vi "ReadCA.vi"(0 "CA":T2(array[cluster]), 1 "Index":u32) -> (7 "square":T1)   [LabVIEW 2020]
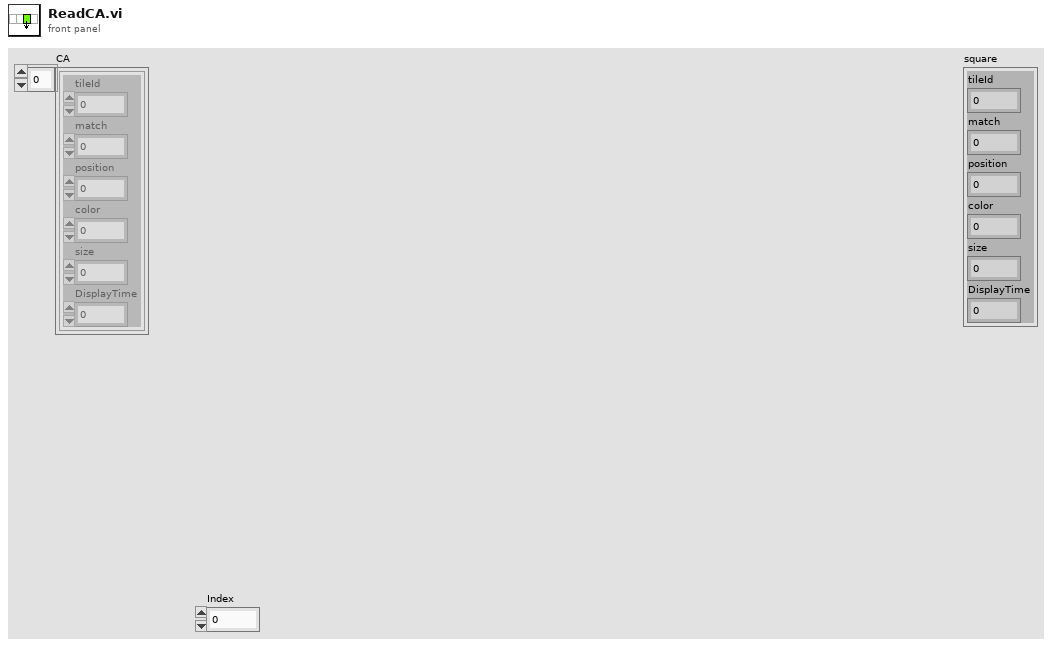
[diagram p1: front panel]
types:
  T1 = cluster{"tileId":i32, "match":i32, "position":i32, "color":u32, "size":i32, "DisplayTime":i32}
  T2 = cluster{"tileId":i32, "match":i32, "position":i32, "color":u32, "size":i32, "DisplayTime":i32}[]
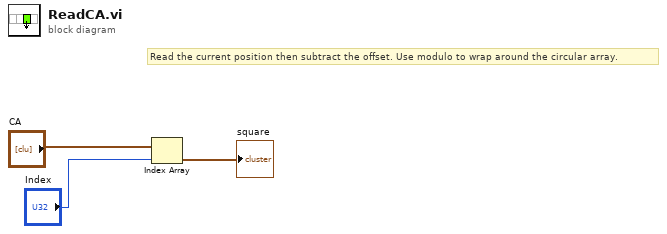
[diagram p0: block diagram]
diagram:
  # "Read the current position then subtract the offset. Use modulo to wrap around the circular array."
  n1 = Index Array(array="CA", index="Index") -> (element=→"square":T1)
